vi "Stats_File_Name_String.vi"(8 "String":string, 10 "N":i32, 11 "TestFreq":i32) -> (2 "Output string":string)   [LabVIEW 2022 SP3]
panel:
  out "FreqStr":string
  out "StartString":string
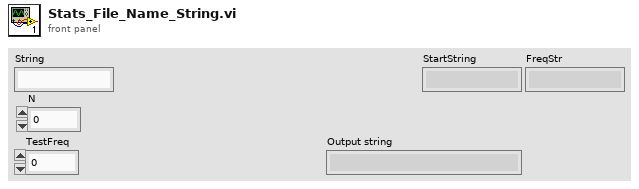
[diagram p1: front panel]
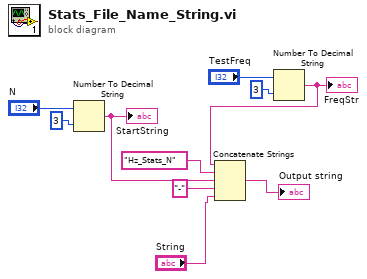
[diagram p0: block diagram]
diagram:
  n1 = Number To Decimal String(number="N", width (-)=i16 3) -> (decimal integer string=w6:string)
  "StartString" <- w6
  n2 = Number To Decimal String(number="TestFreq", width (-)=i16 3) -> (decimal integer string=w2:string)
  "FreqStr" <- w2
  n3 = Concatenate Strings(w2, "Hz_Stats_N" ("string"), w6, "-" ("string"), "String") -> (→"Output string":string)
